vi "Read Config.vi"(8 "error in (no error)":errorcluster, 11 "CsvReportPlugin in":refnum<class "CsvReportPlugin.lvclass">) -> (0 "error out":errorcluster, 2 "Config":variant, 3 "CsvReportPlugin out":refnum<class "CsvReportPlugin.lvclass">)   [LabVIEW 2015, in "CsvReportPlugin.lvclass"]
uses:
  CsvReportPlugin.lvclass
  CsvReportPlugin.lvclass/CsvReportPlugin.ctl
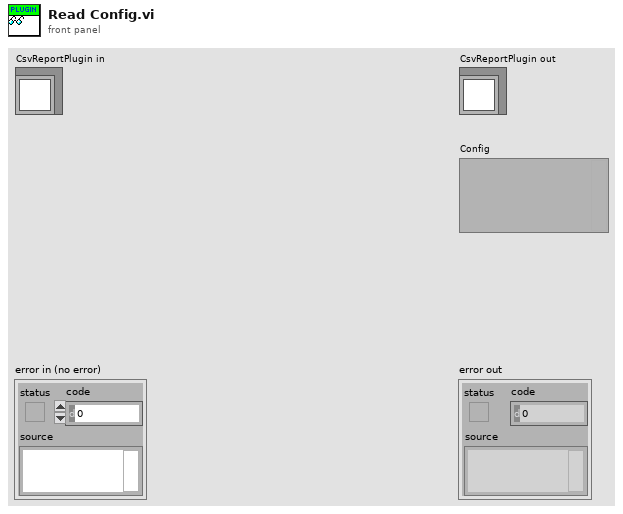
[diagram p1: front panel]
types:
  T1 = cluster{"Enable":bool, "Report Folder":string, "Skip Error Result":bool}
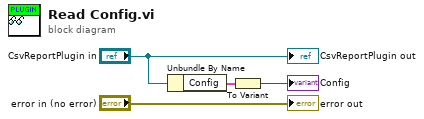
[diagram p0: block diagram]
diagram:
  n1 = Unbundle By Name("CsvReportPlugin in") -> ("Config"=w4:T1)
  n2 = To Variant(anything=w4) -> (Variant=→"Config":variant)
  "error out" <- "error in (no error)"
  "CsvReportPlugin out" <- "CsvReportPlugin in"
